vi "PianoTest 24 channel.vi"() -> ()   [LabVIEW 2013]
uses:
  <vilib>/rvi/Emulation/niFpgaSctlEmulationGetInTimedLoop.vi
  <vilib>/rvi/Emulation/niFpgaEmulationReportErrorSimple.vi
  <vilib>/rvi/Emulation/niFpgaGetClockAttributes.vi
  <vilib>/rvi/eio/common/nirviEmuTemplateMethod_errors.vi
  <vilib>/rvi/Emulation/niFpgaCriticalErrorInLSC.vi
  <vilib>/eio/EIONode/EIONode.xnode
panel:
  in  "PWM1 Period (us)":fxp<+/-,20,16>=130.0
  in  "PWM1 Duty Cycle %":fxp<+/-,20,16>=100.0
  in  "Play":bool
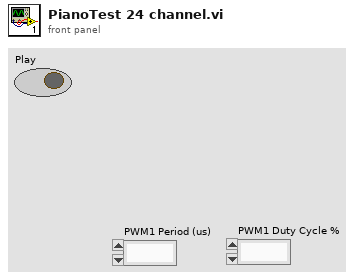
[diagram p1: front panel]
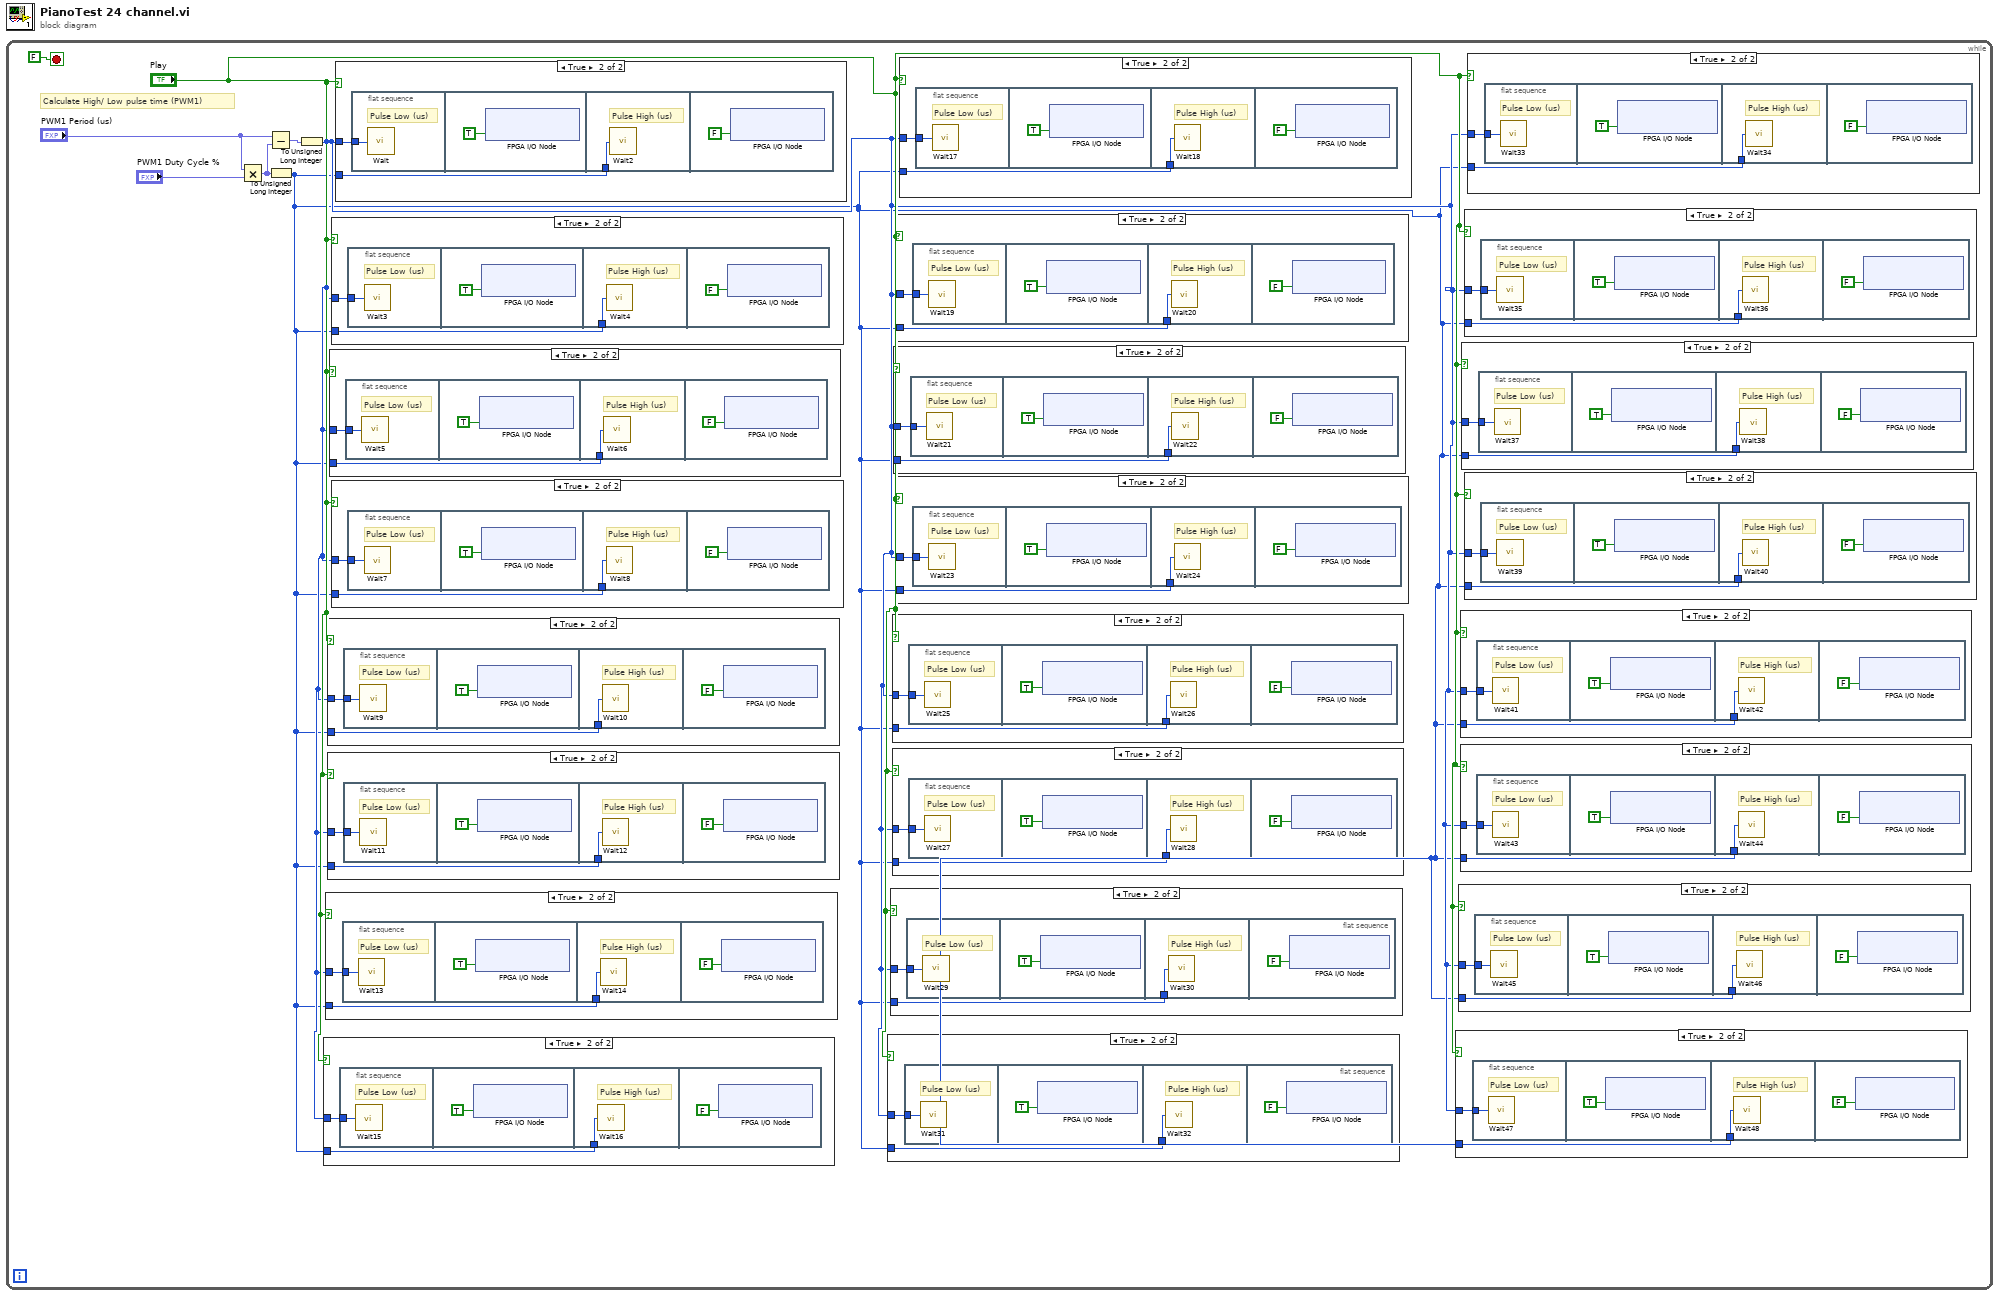
[diagram p0: block diagram]
diagram:
  n1 = while {
    stop <- FALSE stop-if-true
    # "Calculate High/ Low pulse time (PWM1)"
    n2 = Multiply(x="PWM1 Period (us)", y="PWM1 Duty Cycle %") -> (x*y=w7:fxp<+/-,40,32>)
    n3 = Subtract(x="PWM1 Period (us)", y=w7) -> (x-y=w4:fxp<+/-,40,32>)
    n4 = To Unsigned Long Integer(number=w7) -> (unsigned 32bit integer=w1:u32)
    n5 = To Unsigned Long Integer(number=w4) -> (unsigned 32bit integer=w2:u32)
    n6 = case shown="True" "Play" {
      tunnel: w1 -> [_ w106]
      tunnel: w2 -> [_ w105]
      frame False {
      }
      frame True {
        n7 = flat-sequence {
          tunnel: w105 -> [w107]
          tunnel: w106 -> [w109]
          frame #0 {
            # "Pulse Low (us)"
            n8 = call "Wait15"("Count(uSec)"=w107) -> ()  [unwired: 1 out]
          }
          frame #1 {
            n9 = xnode "FPGA I/O Node"("Mod1/DO7"=TRUE ("PWM 1T")) -> ()  [unwired: 1 in, 1 out]
          }
          frame #2 {
            # "Pulse High (us)"
            n10 = call "Wait16"("Count(uSec)"=w109) -> ()  [unwired: 1 out]
          }
          frame #3 {
            n11 = xnode "FPGA I/O Node"("Mod1/DO7"=FALSE ("PWM 1T")) -> ()  [unwired: 1 in, 1 out]
          }
        }
      }
    }
    n12 = case shown="True" "Play" {
      tunnel: w1 -> [_ w112]
      tunnel: w2 -> [_ w111]
      frame False {
      }
      frame True {
        n13 = flat-sequence {
          tunnel: w111 -> [w113]
          tunnel: w112 -> [w115]
          frame #0 {
            # "Pulse Low (us)"
            n14 = call "Wait13"("Count(uSec)"=w113) -> ()  [unwired: 1 out]
          }
          frame #1 {
            n15 = xnode "FPGA I/O Node"("Mod1/DO6"=TRUE ("PWM 1T")) -> ()  [unwired: 1 in, 1 out]
          }
          frame #2 {
            # "Pulse High (us)"
            n16 = call "Wait14"("Count(uSec)"=w115) -> ()  [unwired: 1 out]
          }
          frame #3 {
            n17 = xnode "FPGA I/O Node"("Mod1/DO6"=FALSE ("PWM 1T")) -> ()  [unwired: 1 in, 1 out]
          }
        }
      }
    }
    n18 = case shown="True" "Play" {
      tunnel: w1 -> [_ w124]
      tunnel: w2 -> [_ w123]
      frame False {
      }
      frame True {
        n19 = flat-sequence {
          tunnel: w123 -> [w125]
          tunnel: w124 -> [w127]
          frame #0 {
            # "Pulse Low (us)"
            n20 = call "Wait9"("Count(uSec)"=w125) -> ()  [unwired: 1 out]
          }
          frame #1 {
            n21 = xnode "FPGA I/O Node"("Mod1/DO4"=TRUE ("PWM 1T")) -> ()  [unwired: 1 in, 1 out]
          }
          frame #2 {
            # "Pulse High (us)"
            n22 = call "Wait10"("Count(uSec)"=w127) -> ()  [unwired: 1 out]
          }
          frame #3 {
            n23 = xnode "FPGA I/O Node"("Mod1/DO4"=FALSE ("PWM 1T")) -> ()  [unwired: 1 in, 1 out]
          }
        }
      }
    }
    n24 = case shown="True" "Play" {
      tunnel: w1 -> [_ w118]
      tunnel: w2 -> [_ w117]
      frame False {
      }
      frame True {
        n25 = flat-sequence {
          tunnel: w117 -> [w119]
          tunnel: w118 -> [w121]
          frame #0 {
            # "Pulse Low (us)"
            n26 = call "Wait11"("Count(uSec)"=w119) -> ()  [unwired: 1 out]
          }
          frame #1 {
            n27 = xnode "FPGA I/O Node"("Mod1/DO5"=TRUE ("PWM 1T")) -> ()  [unwired: 1 in, 1 out]
          }
          frame #2 {
            # "Pulse High (us)"
            n28 = call "Wait12"("Count(uSec)"=w121) -> ()  [unwired: 1 out]
          }
          frame #3 {
            n29 = xnode "FPGA I/O Node"("Mod1/DO5"=FALSE ("PWM 1T")) -> ()  [unwired: 1 in, 1 out]
          }
        }
      }
    }
    n30 = case shown="True" "Play" {
      tunnel: w1 -> [_ w136]
      tunnel: w2 -> [_ w135]
      frame False {
      }
      frame True {
        n31 = flat-sequence {
          tunnel: w135 -> [w137]
          tunnel: w136 -> [w139]
          frame #0 {
            # "Pulse Low (us)"
            n32 = call "Wait5"("Count(uSec)"=w137) -> ()  [unwired: 1 out]
          }
          frame #1 {
            n33 = xnode "FPGA I/O Node"("Mod1/DO2"=TRUE ("PWM 1T")) -> ()  [unwired: 1 in, 1 out]
          }
          frame #2 {
            # "Pulse High (us)"
            n34 = call "Wait6"("Count(uSec)"=w139) -> ()  [unwired: 1 out]
          }
          frame #3 {
            n35 = xnode "FPGA I/O Node"("Mod1/DO2"=FALSE ("PWM 1T")) -> ()  [unwired: 1 in, 1 out]
          }
        }
      }
    }
    n36 = case shown="True" "Play" {
      tunnel: w1 -> [_ w142]
      tunnel: w2 -> [_ w141]
      frame False {
      }
      frame True {
        n37 = flat-sequence {
          tunnel: w141 -> [w143]
          tunnel: w142 -> [w145]
          frame #0 {
            # "Pulse Low (us)"
            n38 = call "Wait3"("Count(uSec)"=w143) -> ()  [unwired: 1 out]
          }
          frame #1 {
            n39 = xnode "FPGA I/O Node"("Mod1/DO1"=TRUE ("PWM 1T")) -> ()  [unwired: 1 in, 1 out]
          }
          frame #2 {
            # "Pulse High (us)"
            n40 = call "Wait4"("Count(uSec)"=w145) -> ()  [unwired: 1 out]
          }
          frame #3 {
            n41 = xnode "FPGA I/O Node"("Mod1/DO1"=FALSE ("PWM 1T")) -> ()  [unwired: 1 in, 1 out]
          }
        }
      }
    }
    n42 = case shown="True" "Play" {
      tunnel: w1 -> [_ w130]
      tunnel: w2 -> [_ w129]
      frame False {
      }
      frame True {
        n43 = flat-sequence {
          tunnel: w129 -> [w131]
          tunnel: w130 -> [w133]
          frame #0 {
            # "Pulse Low (us)"
            n44 = call "Wait7"("Count(uSec)"=w131) -> ()  [unwired: 1 out]
          }
          frame #1 {
            n45 = xnode "FPGA I/O Node"("Mod1/DO3"=TRUE ("PWM 1T")) -> ()  [unwired: 1 in, 1 out]
          }
          frame #2 {
            # "Pulse High (us)"
            n46 = call "Wait8"("Count(uSec)"=w133) -> ()  [unwired: 1 out]
          }
          frame #3 {
            n47 = xnode "FPGA I/O Node"("Mod1/DO3"=FALSE ("PWM 1T")) -> ()  [unwired: 1 in, 1 out]
          }
        }
      }
    }
    n48 = case shown="True" "Play" {
      tunnel: w1 -> [_ w148]
      tunnel: w2 -> [_ w147]
      frame False {
      }
      frame True {
        n49 = flat-sequence {
          tunnel: w147 -> [w149]
          tunnel: w148 -> [w151]
          frame #0 {
            # "Pulse Low (us)"
            n50 = call "Wait"("Count(uSec)"=w149) -> ()  [unwired: 1 out]
          }
          frame #1 {
            n51 = xnode "FPGA I/O Node"("Mod1/DO0"=TRUE ("PWM 1T")) -> ()  [unwired: 1 in, 1 out]
          }
          frame #2 {
            # "Pulse High (us)"
            n52 = call "Wait2"("Count(uSec)"=w151) -> ()  [unwired: 1 out]
          }
          frame #3 {
            n53 = xnode "FPGA I/O Node"("Mod1/DO0"=FALSE ("PWM 1T")) -> ()  [unwired: 1 in, 1 out]
          }
        }
      }
    }
    n54 = case shown="True" "Play" {
      tunnel: w1 -> [_ w58]
      tunnel: w2 -> [_ w57]
      frame False {
      }
      frame True {
        n55 = flat-sequence {
          tunnel: w57 -> [w59]
          tunnel: w58 -> [w61]
          frame #0 {
            # "Pulse Low (us)"
            n56 = call "Wait31"("Count(uSec)"=w59) -> ()  [unwired: 1 out]
          }
          frame #1 {
            n57 = xnode "FPGA I/O Node"("Mod1/DO15"=TRUE ("PWM 1T")) -> ()  [unwired: 1 in, 1 out]
          }
          frame #2 {
            # "Pulse High (us)"
            n58 = call "Wait32"("Count(uSec)"=w61) -> ()  [unwired: 1 out]
          }
          frame #3 {
            n59 = xnode "FPGA I/O Node"("Mod1/DO15"=FALSE ("PWM 1T")) -> ()  [unwired: 1 in, 1 out]
          }
        }
      }
    }
    n60 = case shown="True" "Play" {
      tunnel: w1 -> [_ w64]
      tunnel: w2 -> [_ w63]
      frame False {
      }
      frame True {
        n61 = flat-sequence {
          tunnel: w63 -> [w65]
          tunnel: w64 -> [w67]
          frame #0 {
            # "Pulse Low (us)"
            n62 = call "Wait29"("Count(uSec)"=w65) -> ()  [unwired: 1 out]
          }
          frame #1 {
            n63 = xnode "FPGA I/O Node"("Mod1/DO14"=TRUE ("PWM 1T")) -> ()  [unwired: 1 in, 1 out]
          }
          frame #2 {
            # "Pulse High (us)"
            n64 = call "Wait30"("Count(uSec)"=w67) -> ()  [unwired: 1 out]
          }
          frame #3 {
            n65 = xnode "FPGA I/O Node"("Mod1/DO14"=FALSE ("PWM 1T")) -> ()  [unwired: 1 in, 1 out]
          }
        }
      }
    }
    n66 = case shown="True" "Play" {
      tunnel: w1 -> [_ w76]
      tunnel: w2 -> [_ w75]
      frame False {
      }
      frame True {
        n67 = flat-sequence {
          tunnel: w75 -> [w77]
          tunnel: w76 -> [w79]
          frame #0 {
            # "Pulse Low (us)"
            n68 = call "Wait25"("Count(uSec)"=w77) -> ()  [unwired: 1 out]
          }
          frame #1 {
            n69 = xnode "FPGA I/O Node"("Mod1/DO12"=TRUE ("PWM 1T")) -> ()  [unwired: 1 in, 1 out]
          }
          frame #2 {
            # "Pulse High (us)"
            n70 = call "Wait26"("Count(uSec)"=w79) -> ()  [unwired: 1 out]
          }
          frame #3 {
            n71 = xnode "FPGA I/O Node"("Mod1/DO12"=FALSE ("PWM 1T")) -> ()  [unwired: 1 in, 1 out]
          }
        }
      }
    }
    n72 = case shown="True" "Play" {
      tunnel: w1 -> [_ w70]
      tunnel: w2 -> [_ w69]
      frame False {
      }
      frame True {
        n73 = flat-sequence {
          tunnel: w69 -> [w71]
          tunnel: w70 -> [w73]
          frame #0 {
            # "Pulse Low (us)"
            n74 = call "Wait27"("Count(uSec)"=w71) -> ()  [unwired: 1 out]
          }
          frame #1 {
            n75 = xnode "FPGA I/O Node"("Mod1/DO13"=TRUE ("PWM 1T")) -> ()  [unwired: 1 in, 1 out]
          }
          frame #2 {
            # "Pulse High (us)"
            n76 = call "Wait28"("Count(uSec)"=w73) -> ()  [unwired: 1 out]
          }
          frame #3 {
            n77 = xnode "FPGA I/O Node"("Mod1/DO13"=FALSE ("PWM 1T")) -> ()  [unwired: 1 in, 1 out]
          }
        }
      }
    }
    n78 = case shown="True" "Play" {
      tunnel: w1 -> [_ w88]
      tunnel: w2 -> [_ w87]
      frame False {
      }
      frame True {
        n79 = flat-sequence {
          tunnel: w87 -> [w89]
          tunnel: w88 -> [w91]
          frame #0 {
            # "Pulse Low (us)"
            n80 = call "Wait21"("Count(uSec)"=w89) -> ()  [unwired: 1 out]
          }
          frame #1 {
            n81 = xnode "FPGA I/O Node"("Mod1/DO10"=TRUE ("PWM 1T")) -> ()  [unwired: 1 in, 1 out]
          }
          frame #2 {
            # "Pulse High (us)"
            n82 = call "Wait22"("Count(uSec)"=w91) -> ()  [unwired: 1 out]
          }
          frame #3 {
            n83 = xnode "FPGA I/O Node"("Mod1/DO10"=FALSE ("PWM 1T")) -> ()  [unwired: 1 in, 1 out]
          }
        }
      }
    }
    n84 = case shown="True" "Play" {
      tunnel: w1 -> [_ w94]
      tunnel: w2 -> [_ w93]
      frame False {
      }
      frame True {
        n85 = flat-sequence {
          tunnel: w93 -> [w95]
          tunnel: w94 -> [w97]
          frame #0 {
            # "Pulse Low (us)"
            n86 = call "Wait19"("Count(uSec)"=w95) -> ()  [unwired: 1 out]
          }
          frame #1 {
            n87 = xnode "FPGA I/O Node"("Mod1/DO9"=TRUE ("PWM 1T")) -> ()  [unwired: 1 in, 1 out]
          }
          frame #2 {
            # "Pulse High (us)"
            n88 = call "Wait20"("Count(uSec)"=w97) -> ()  [unwired: 1 out]
          }
          frame #3 {
            n89 = xnode "FPGA I/O Node"("Mod1/DO9"=FALSE ("PWM 1T")) -> ()  [unwired: 1 in, 1 out]
          }
        }
      }
    }
    n90 = case shown="True" "Play" {
      tunnel: w1 -> [_ w82]
      tunnel: w2 -> [_ w81]
      frame False {
      }
      frame True {
        n91 = flat-sequence {
          tunnel: w81 -> [w83]
          tunnel: w82 -> [w85]
          frame #0 {
            # "Pulse Low (us)"
            n92 = call "Wait23"("Count(uSec)"=w83) -> ()  [unwired: 1 out]
          }
          frame #1 {
            n93 = xnode "FPGA I/O Node"("Mod1/DO11"=TRUE ("PWM 1T")) -> ()  [unwired: 1 in, 1 out]
          }
          frame #2 {
            # "Pulse High (us)"
            n94 = call "Wait24"("Count(uSec)"=w85) -> ()  [unwired: 1 out]
          }
          frame #3 {
            n95 = xnode "FPGA I/O Node"("Mod1/DO11"=FALSE ("PWM 1T")) -> ()  [unwired: 1 in, 1 out]
          }
        }
      }
    }
    n96 = case shown="True" "Play" {
      tunnel: w1 -> [_ w100]
      tunnel: w2 -> [_ w99]
      frame False {
      }
      frame True {
        n97 = flat-sequence {
          tunnel: w99 -> [w101]
          tunnel: w100 -> [w103]
          frame #0 {
            # "Pulse Low (us)"
            n98 = call "Wait17"("Count(uSec)"=w101) -> ()  [unwired: 1 out]
          }
          frame #1 {
            n99 = xnode "FPGA I/O Node"("Mod1/DO8"=TRUE ("PWM 1T")) -> ()  [unwired: 1 in, 1 out]
          }
          frame #2 {
            # "Pulse High (us)"
            n100 = call "Wait18"("Count(uSec)"=w103) -> ()  [unwired: 1 out]
          }
          frame #3 {
            n101 = xnode "FPGA I/O Node"("Mod1/DO8"=FALSE ("PWM 1T")) -> ()  [unwired: 1 in, 1 out]
          }
        }
      }
    }
    n102 = case shown="True" "Play" {
      tunnel: w1 -> [_ w10]
      tunnel: w2 -> [_ w9]
      frame False {
      }
      frame True {
        n103 = flat-sequence {
          tunnel: w9 -> [w11]
          tunnel: w10 -> [w13]
          frame #0 {
            # "Pulse Low (us)"
            n104 = call "Wait47"("Count(uSec)"=w11) -> ()  [unwired: 1 out]
          }
          frame #1 {
            n105 = xnode "FPGA I/O Node"("Mod1/DO23"=TRUE ("PWM 1T")) -> ()  [unwired: 1 in, 1 out]
          }
          frame #2 {
            # "Pulse High (us)"
            n106 = call "Wait48"("Count(uSec)"=w13) -> ()  [unwired: 1 out]
          }
          frame #3 {
            n107 = xnode "FPGA I/O Node"("Mod1/DO23"=FALSE ("PWM 1T")) -> ()  [unwired: 1 in, 1 out]
          }
        }
      }
    }
    n108 = case shown="True" "Play" {
      tunnel: w1 -> [_ w16]
      tunnel: w2 -> [_ w15]
      frame False {
      }
      frame True {
        n109 = flat-sequence {
          tunnel: w15 -> [w17]
          tunnel: w16 -> [w19]
          frame #0 {
            # "Pulse Low (us)"
            n110 = call "Wait45"("Count(uSec)"=w17) -> ()  [unwired: 1 out]
          }
          frame #1 {
            n111 = xnode "FPGA I/O Node"("Mod1/DO22"=TRUE ("PWM 1T")) -> ()  [unwired: 1 in, 1 out]
          }
          frame #2 {
            # "Pulse High (us)"
            n112 = call "Wait46"("Count(uSec)"=w19) -> ()  [unwired: 1 out]
          }
          frame #3 {
            n113 = xnode "FPGA I/O Node"("Mod1/DO22"=FALSE ("PWM 1T")) -> ()  [unwired: 1 in, 1 out]
          }
        }
      }
    }
    n114 = case shown="True" "Play" {
      tunnel: w1 -> [_ w28]
      tunnel: w2 -> [_ w27]
      frame False {
      }
      frame True {
        n115 = flat-sequence {
          tunnel: w27 -> [w29]
          tunnel: w28 -> [w31]
          frame #0 {
            # "Pulse Low (us)"
            n116 = call "Wait41"("Count(uSec)"=w29) -> ()  [unwired: 1 out]
          }
          frame #1 {
            n117 = xnode "FPGA I/O Node"("Mod1/DO20"=TRUE ("PWM 1T")) -> ()  [unwired: 1 in, 1 out]
          }
          frame #2 {
            # "Pulse High (us)"
            n118 = call "Wait42"("Count(uSec)"=w31) -> ()  [unwired: 1 out]
          }
          frame #3 {
            n119 = xnode "FPGA I/O Node"("Mod1/DO20"=FALSE ("PWM 1T")) -> ()  [unwired: 1 in, 1 out]
          }
        }
      }
    }
    n120 = case shown="True" "Play" {
      tunnel: w1 -> [_ w22]
      tunnel: w2 -> [_ w21]
      frame False {
      }
      frame True {
        n121 = flat-sequence {
          tunnel: w21 -> [w23]
          tunnel: w22 -> [w25]
          frame #0 {
            # "Pulse Low (us)"
            n122 = call "Wait43"("Count(uSec)"=w23) -> ()  [unwired: 1 out]
          }
          frame #1 {
            n123 = xnode "FPGA I/O Node"("Mod1/DO21"=TRUE ("PWM 1T")) -> ()  [unwired: 1 in, 1 out]
          }
          frame #2 {
            # "Pulse High (us)"
            n124 = call "Wait44"("Count(uSec)"=w25) -> ()  [unwired: 1 out]
          }
          frame #3 {
            n125 = xnode "FPGA I/O Node"("Mod1/DO21"=FALSE ("PWM 1T")) -> ()  [unwired: 1 in, 1 out]
          }
        }
      }
    }
    n126 = case shown="True" "Play" {
      tunnel: w1 -> [_ w40]
      tunnel: w2 -> [_ w39]
      frame False {
      }
      frame True {
        n127 = flat-sequence {
          tunnel: w39 -> [w41]
          tunnel: w40 -> [w43]
          frame #0 {
            # "Pulse Low (us)"
            n128 = call "Wait37"("Count(uSec)"=w41) -> ()  [unwired: 1 out]
          }
          frame #1 {
            n129 = xnode "FPGA I/O Node"("Mod1/DO18"=TRUE ("PWM 1T")) -> ()  [unwired: 1 in, 1 out]
          }
          frame #2 {
            # "Pulse High (us)"
            n130 = call "Wait38"("Count(uSec)"=w43) -> ()  [unwired: 1 out]
          }
          frame #3 {
            n131 = xnode "FPGA I/O Node"("Mod1/DO18"=FALSE ("PWM 1T")) -> ()  [unwired: 1 in, 1 out]
          }
        }
      }
    }
    n132 = case shown="True" "Play" {
      tunnel: w1 -> [_ w46]
      tunnel: w2 -> [_ w45]
      frame False {
      }
      frame True {
        n133 = flat-sequence {
          tunnel: w45 -> [w47]
          tunnel: w46 -> [w49]
          frame #0 {
            # "Pulse Low (us)"
            n134 = call "Wait35"("Count(uSec)"=w47) -> ()  [unwired: 1 out]
          }
          frame #1 {
            n135 = xnode "FPGA I/O Node"("Mod1/DO17"=TRUE ("PWM 1T")) -> ()  [unwired: 1 in, 1 out]
          }
          frame #2 {
            # "Pulse High (us)"
            n136 = call "Wait36"("Count(uSec)"=w49) -> ()  [unwired: 1 out]
          }
          frame #3 {
            n137 = xnode "FPGA I/O Node"("Mod1/DO17"=FALSE ("PWM 1T")) -> ()  [unwired: 1 in, 1 out]
          }
        }
      }
    }
    n138 = case shown="True" "Play" {
      tunnel: w1 -> [_ w34]
      tunnel: w2 -> [_ w33]
      frame False {
      }
      frame True {
        n139 = flat-sequence {
          tunnel: w33 -> [w35]
          tunnel: w34 -> [w37]
          frame #0 {
            # "Pulse Low (us)"
            n140 = call "Wait39"("Count(uSec)"=w35) -> ()  [unwired: 1 out]
          }
          frame #1 {
            n141 = xnode "FPGA I/O Node"("Mod1/DO19"=TRUE ("PWM 1T")) -> ()  [unwired: 1 in, 1 out]
          }
          frame #2 {
            # "Pulse High (us)"
            n142 = call "Wait40"("Count(uSec)"=w37) -> ()  [unwired: 1 out]
          }
          frame #3 {
            n143 = xnode "FPGA I/O Node"("Mod1/DO19"=FALSE ("PWM 1T")) -> ()  [unwired: 1 in, 1 out]
          }
        }
      }
    }
    n144 = case shown="True" "Play" {
      tunnel: w1 -> [_ w52]
      tunnel: w2 -> [_ w51]
      frame False {
      }
      frame True {
        n145 = flat-sequence {
          tunnel: w51 -> [w53]
          tunnel: w52 -> [w55]
          frame #0 {
            # "Pulse Low (us)"
            n146 = call "Wait33"("Count(uSec)"=w53) -> ()  [unwired: 1 out]
          }
          frame #1 {
            n147 = xnode "FPGA I/O Node"("Mod1/DO16"=TRUE ("PWM 1T")) -> ()  [unwired: 1 in, 1 out]
          }
          frame #2 {
            # "Pulse High (us)"
            n148 = call "Wait34"("Count(uSec)"=w55) -> ()  [unwired: 1 out]
          }
          frame #3 {
            n149 = xnode "FPGA I/O Node"("Mod1/DO16"=FALSE ("PWM 1T")) -> ()  [unwired: 1 in, 1 out]
          }
        }
      }
    }
  }
